vi "getPiezowaveformarray.vi"(7 "planes or zigzag":bool, 8 "pixel.num":i32=10000, 9 "frames.per.z.cycle":dbl=15.0, 10 "total.z.distance":dbl=100.0, 11 "piezo scale factor":dbl=0.025) -> (3 "Array":dbl[](array[numeric]))   [LabVIEW 2012]
panel:
  out "Waveform Graph":dbl[](graph)
  out "min value":dbl
  out "max value":dbl
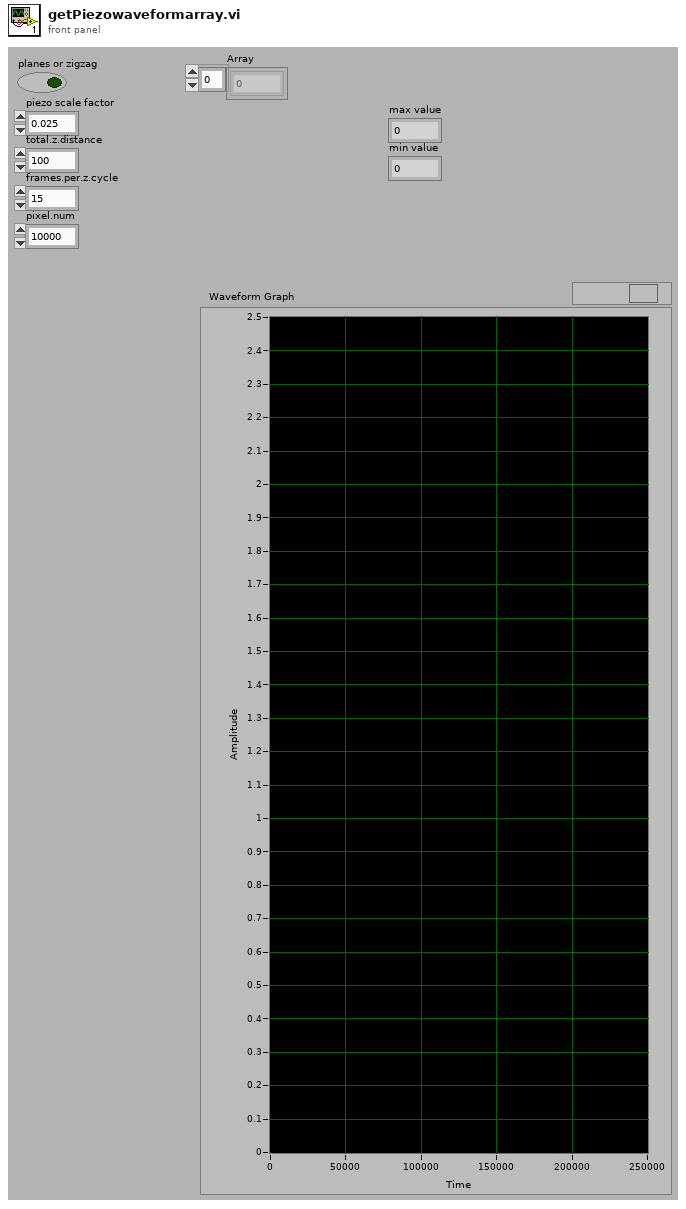
[diagram p1: front panel]
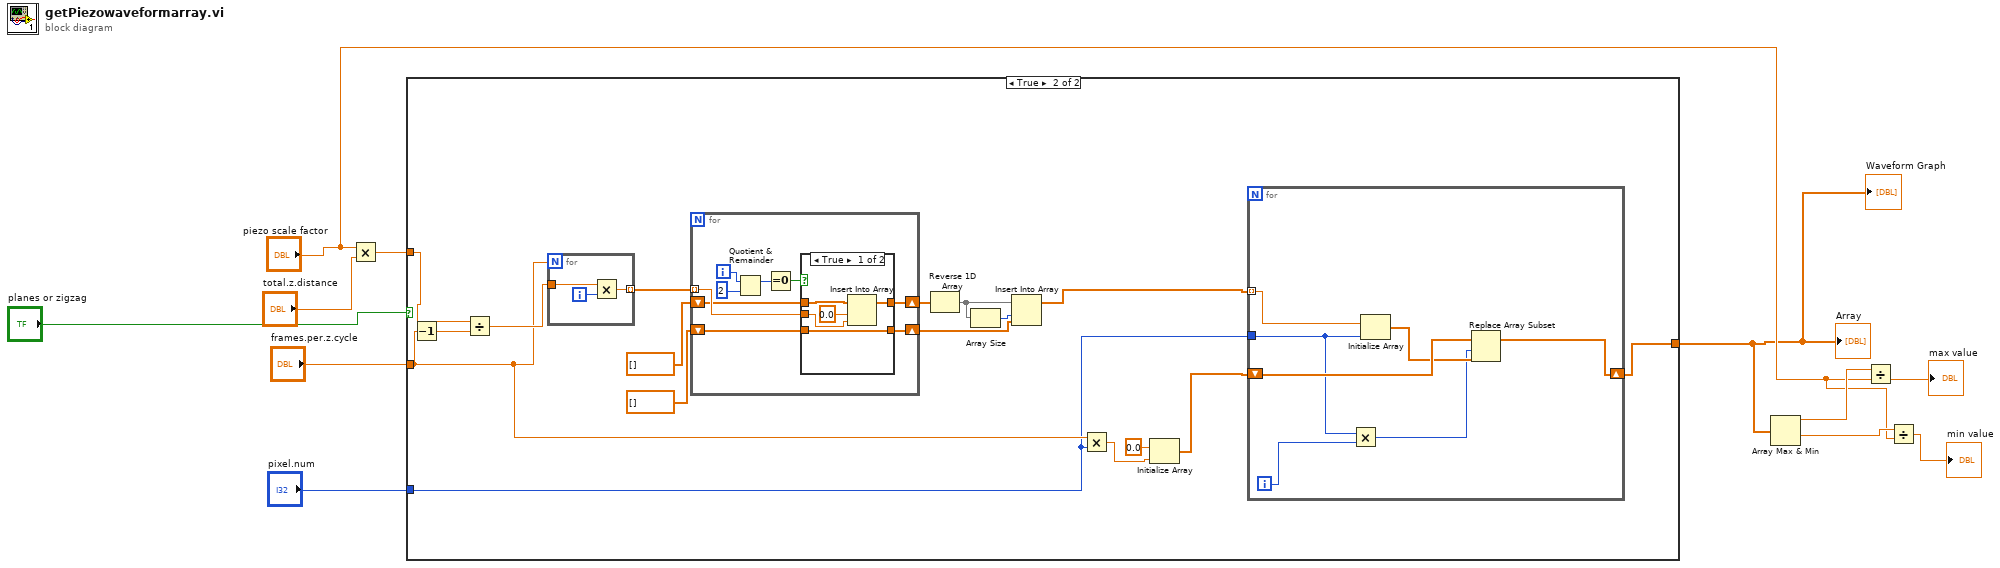
[diagram p0: block diagram]
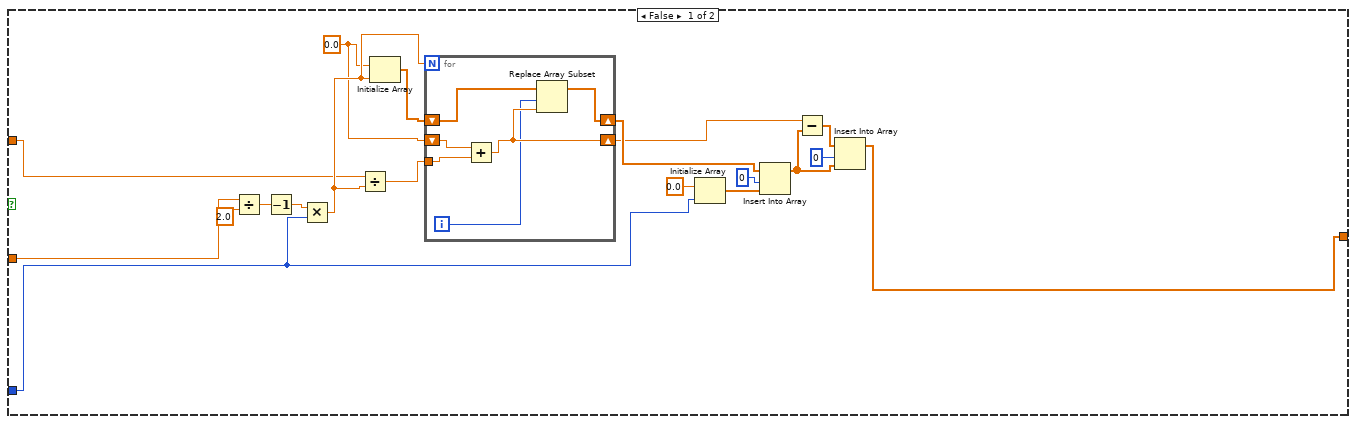
[diagram p2: hidden frame]
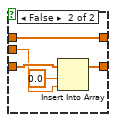
[diagram p3: hidden frame]
diagram:
  n1 = Multiply(x="piezo scale factor", y="total.z.distance") -> (x*y=w10:dbl)
  n2 = case shown="True" "planes or zigzag" {
    tunnel: [w12 w41] -> w1
    tunnel: w10 -> [w15 w40]
    tunnel: "frames.per.z.cycle" -> [w14 w39]
    tunnel: "pixel.num" -> [w13 w38]
    frame False {
      w24 = 0.0 ("element")
      n3 = Divide(x=w14, y=2.0) -> (x/y=w29:dbl)
      n4 = Decrement(x=w29) -> (x-1=w28:dbl)
      n5 = Multiply(x=w28, y=w13) -> (x*y=w25:dbl)
      n6 = Divide(x=w15, y=w25) -> (x/y=w26:dbl)
      n7 = Initialize Array(w24, w25) -> (w27:dbl[])
      n8 = for {
        N: w25 -> [_]
        shift-right: [w33] -> w17
        shift-left: w27 -> [w34]
        tunnel: w26 -> [w35]
        shift-right: [w32] -> w16
        shift-left: w24 -> [w36]
        i -> [w31]
        n9 = Add(x=w36, y=w35) -> (x+y=w32:dbl)
        n10 = Replace Array Subset(array=w34, new element=w32, index=w31) -> (w33:dbl[])
      }
      n11 = Initialize Array(0.0 ("element"), w13) -> (w19:dbl[])
      n12 = Insert Into Array(array=w17, index=0, new element=w19) -> (w23:dbl[])
      n13 = Subtract(x=w16, y=w23) -> (x-y=w22:dbl[])
      n14 = Insert Into Array(array=w22, index=0, new element=w23) -> (w12:dbl[])
    }
    frame True {
      n15 = Decrement(x=w39) -> (x-1=w37:dbl)
      n16 = Divide(x=w40, y=w37) -> (x/y=w53:dbl)
      n17 = for {
        N: w39 -> [_]
        tunnel: w53 -> [w82]
        tunnel: [w80] -> w52 mode=indexing
        i -> [w81]
        n18 = Multiply(x=w82, y=w81) -> (x*y=w80:dbl)
      }
      n19 = for {
        shift-right: [w63] -> w48
        shift-left: dbl[] [] -> [w62]
        shift-right: [w64] -> w47
        shift-left: dbl[] [] -> [w65]
        tunnel: w52 -> [w67] mode=indexing
        i -> [w66]
        n20 = Quotient & Remainder(x=w66, y=2) -> (x-y*floor(x/y)=w61:i32)  [unwired: 1 out]
        n21 = Equal To 0?(x=w61) -> (x = 0?=w68:bool)
        n22 = case shown="True" w68 {
          tunnel: w67 -> [w70 w75]
          tunnel: w65 -> [w74 w76]
          tunnel: [w72 w76] -> w64
          tunnel: [w71 w77] -> w63
          tunnel: w62 -> [w71 w78]
          frame True {
            n23 = Insert Into Array(array=w74, index=0.0 ("new element/subarray"), new element=w70) -> (w72:dbl[])
          }
          frame False {
            n24 = Insert Into Array(array=w78, index=0.0 ("new element/subarray"), new element=w75) -> (w77:dbl[])
          }
        }
      }
      n25 = Reverse 1D Array(array=w47) -> (reversed array=w46:dbl[])
      n26 = Array Size(array=w46) -> (size(s)=w49:i32)
      n27 = Insert Into Array(array=w46, index=w49, new element=w48) -> (w45:dbl[])
      n28 = Multiply(x=w39, y=w38) -> (x*y=w42:dbl)
      n29 = Initialize Array(0.0 ("element"), w42) -> (w43:dbl[])
      n30 = for {
        tunnel: w45 -> [w60] mode=indexing
        shift-right: [w54] -> w41
        shift-left: w43 -> [w59]
        tunnel: w38 -> [w57]
        i -> [w56]
        n31 = Multiply(x=w57, y=w56) -> (x*y=w55:i32)
        n32 = Initialize Array(w60, w57) -> (w58:dbl[])
        n33 = Replace Array Subset(array=w59, new element=w58, index=w55) -> (w54:dbl[])
      }
    }
  }
  "Array" <- w1
  "Waveform Graph" <- w1
  n34 = Array Max & Min(array=w1) -> (max value=w5:dbl, min value=w4:dbl)  [unwired: 2 out]
  n35 = Divide(x=w5, y="piezo scale factor") -> (x/y=→"max value":dbl)
  n36 = Divide(x=w4, y="piezo scale factor") -> (x/y=→"min value":dbl)
